vi "eventHandler.vi"(8 "error in (no error)":errorcluster, 9 ":HWControllerEvents":refnum<class "HWControllerEvents.lvclass">, 10 "ExperimentControlEvents":refnum<class "ExperimentControlEvents.lvclass">, 11 "ExperimentControl in":refnum<class "ExperimentControl.lvclass">) -> (0 "error out":errorcluster, 3 "ExperimentControl out":refnum<class "ExperimentControl.lvclass">)   [LabVIEW 2009, in "Views.lvlib" / "ExperimentControl.lvlib" / "ExperimentControl.lvclass"]
uses:
  ExperimentControl.lvclass
  Events/ExperimentControlEvents.lvclass
  Hal/HWController/HWControllerEvents/HWControllerEvents.lvclass
  ExperimentControl.lvclass/ExperimentControl.ctl
  Events/Event.lvclass
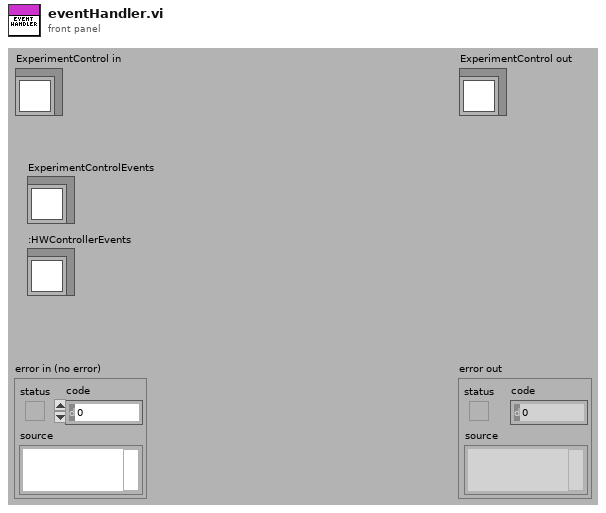
[diagram p1: front panel]
types:
  T1 = enum16{"Ready", "Compiling", "Configured", "Running", "Stopping", "Unresolved Error"}
  T2 = enum16{"close", "stopRunning", "runSingleScript", "runExperiment", "runExperimentScript", "Unregistered", "hasStopped"}
  T3 = cluster{"Array":path[], "Enum":enum16{"runListOnce", "loopOverList"}}
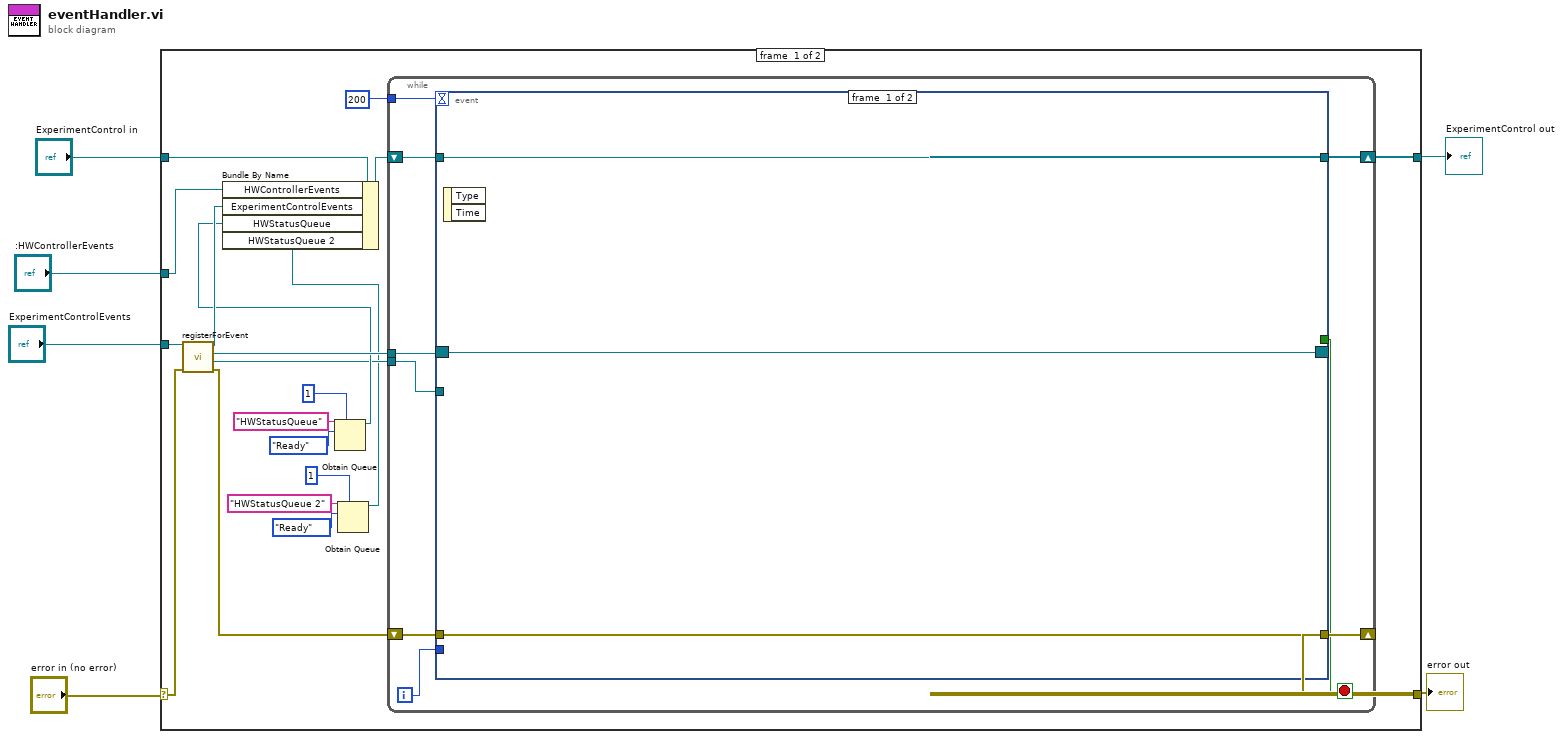
[diagram p0: block diagram]
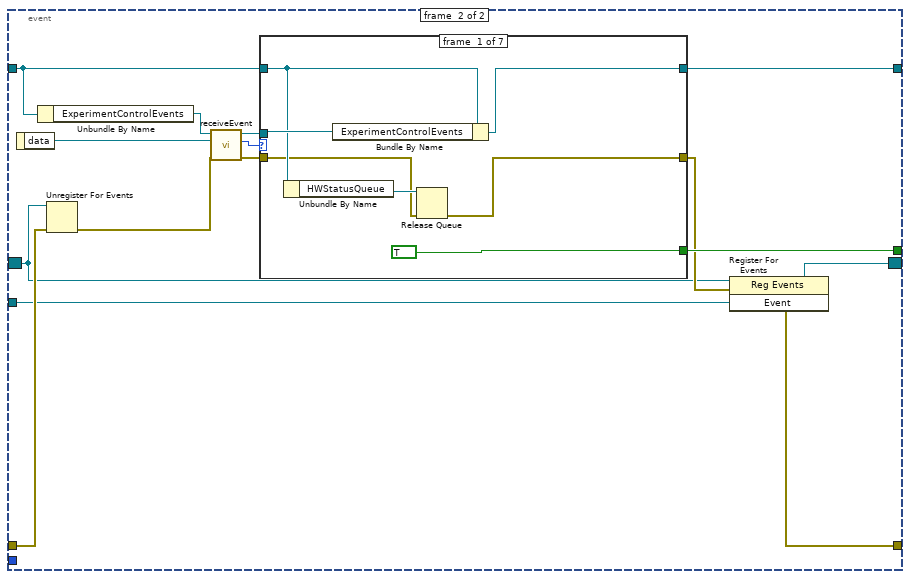
[diagram p2: hidden frame]
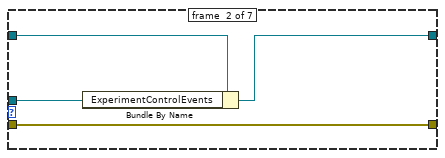
[diagram p3: hidden frame]
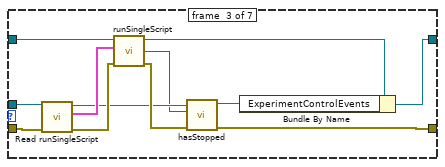
[diagram p4: hidden frame]
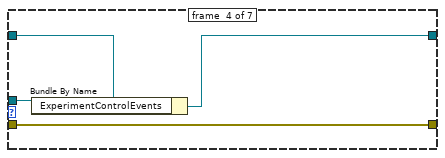
[diagram p5: hidden frame]
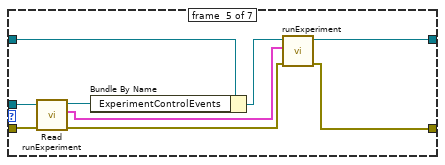
[diagram p6: hidden frame]
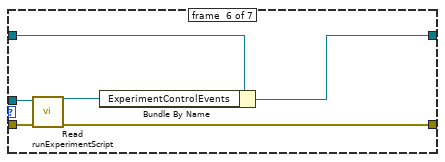
[diagram p7: hidden frame]
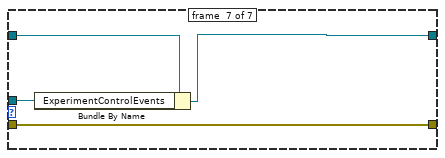
[diagram p8: hidden frame]
diagram:
  n1 = case shown="No Error" "error in (no error)" {
    selector: "error in (no error)" -> [w21 w101]
    tunnel: [w25 w101] -> w5
    tunnel: [w26 w100] -> w1
    tunnel: "ExperimentControl in" -> [w24 w100]
    tunnel: "ExperimentControlEvents" -> [w22 _]
    tunnel: ":HWControllerEvents" -> [w17 _]
    frame #0 {
      n2 = call "registerForEvent.vi"("error in (no error)"=w21, "Event in"=w22) -> ("error out"=w19:errorcluster, "Event"=w11:refnum<user-event>, "Event Registration Refnum"=w20:refnum<event-registration>, "Event out"=w18:refnum<class "ExperimentControlEvents.lvclass">)  [unwired: 6 in]
      n3 = Obtain Queue(max queue size (-1, unlimited)=1, name (unnamed)="HWStatusQueue", element data type=T1."Ready" ("status")) -> (queue out=w12:refnum<queue>)  [unwired: 2 in, 2 out]
      n4 = Obtain Queue(max queue size (-1, unlimited)=1, name (unnamed)="HWStatusQueue 2", element data type=T1."Ready" ("status")) -> (queue out=w7:refnum<queue>)  [unwired: 2 in, 2 out]
      n5 = Bundle By Name(cluster=w24, "HWControllerEvents"=w17, "ExperimentControlEvents"=w18, "HWStatusQueue"=w12, "HWStatusQueue 2"=w7) -> (w23:refnum<class "ExperimentControl.lvclass">)
      n6 = while {
        shift-right: [w32] -> w25
        shift-left: w19 -> [w33]
        shift-right: [w35] -> w26
        shift-left: w23 -> [w34]
        tunnel: w20 -> [w31]
        tunnel: 200 -> [w27]
        tunnel: w11 -> [w28]
        i -> [w29]
        stop <- w30 stop-if-true
        n7 = event shown="[1] <Event>: User Event" {
          selector: w31 -> [w36 w39]
          dyn-events: [w36 w41] -> _
          timeout: w27 -> [_ _]
          tunnel: [w38 w44] -> w35
          tunnel: w34 -> [w38 w48]
          tunnel: w33 -> [w37 w46]
          tunnel: [w37 w40] -> w32
          tunnel: [_ w50] -> w30
          tunnel: w29 -> [_ _]
          tunnel: w28 -> [_ w43]
          event #0 {
            n8 = event-data() -> ()  [unwired: 1 in, 2 out]
          }
          event #1 {
            n9 = event-data() -> ("data"=w52:refnum<class>)  [unwired: 1 in]
            n10 = Unbundle By Name(w48) -> ("ExperimentControlEvents"=w53:refnum<class "ExperimentControlEvents.lvclass">)
            n11 = Unregister For Events(event registration refnum=w39, error in=w46) -> (error out=w45:errorcluster)
            n12 = call "receiveEvent.vi"("error in (no error)"=w45, "data"=w52, "ExperimentControlEvents in"=w53) -> ("error out"=w49:errorcluster, "Enum"=w51:T2, "ExperimentControlEvents out"=w47:refnum<class "ExperimentControlEvents.lvclass">)  [unwired: 6 in]
            n13 = case shown="\"hasStopped\"" w51 {
              tunnel: w47 -> [w58 w62 w74 w79 w89 w92 w98]
              tunnel: [TRUE _ _ _ _ _ _] -> w50
              tunnel: w49 -> [w55 w61 w73 w80 w88 w93 w99]
              tunnel: [w54 w61 w72 w80 w82 w90 w99] -> w42
              tunnel: w48 -> [w57 w64 w70 w78 w86 w95 w97]
              tunnel: [w59 w63 w66 w77 w84 w94 w96] -> w44
              frame #0 {
                n14 = Unbundle By Name(w57) -> ("HWStatusQueue"=w56:refnum<queue>)
                n15 = Bundle By Name(cluster=w57, "ExperimentControlEvents"=w58) -> (w59:refnum<class "ExperimentControl.lvclass">)
                n16 = Release Queue(queue=w56, error in (no error)=w55) -> (error out=w54:errorcluster)  [unwired: 1 in, 2 out]
              }
              frame #1 {
                n17 = Bundle By Name(cluster=w64, "ExperimentControlEvents"=w62) -> (w63:refnum<class "ExperimentControl.lvclass">)
              }
              frame #2 {
                n18 = call "Read runSingleScript.vi"("error in (no error)"=w73, "ExperimentControlEvents in"=w74) -> ("error out"=w76:errorcluster, "runSingleScript"=w75:cluster{"Path":path, "HWLoop":bool}, "ExperimentControlEvents out"=w69:refnum<class "ExperimentControlEvents.lvclass">)  [unwired: 7 in]
                n19 = call "runSingleScript.vi"("error in (no error)"=w76, "runSingleScript"=w75, "ExperimentControl in"=w70) -> ("error out"=w71:errorcluster, "stoppedByUser"=w65:bool, "ExperimentControl out"=w67:refnum<class "ExperimentControl.lvclass">)  [unwired: 5 in, 1 out]
                n20 = call "hasStopped.vi"("error in (no error)"=w71, "stoppedByUser"=w65, "ExperimentControlEvents in"=w69) -> ("error out"=w72:errorcluster, "ExperimentControlEvents out"=w68:refnum<class "ExperimentControlEvents.lvclass">)  [unwired: 7 in]
                n21 = Bundle By Name(cluster=w67, "ExperimentControlEvents"=w68) -> (w66:refnum<class "ExperimentControl.lvclass">)
              }
              frame #3 {
                n22 = Bundle By Name(cluster=w78, "ExperimentControlEvents"=w79) -> (w77:refnum<class "ExperimentControl.lvclass">)
              }
              frame #4 {
                n23 = call "Read runExperiment.vi"("error in (no error)"=w88, "ExperimentControlEvents in"=w89) -> ("error out"=w83:errorcluster, "runExperiment"=w81:T3, "ExperimentControlEvents out"=w87:refnum<class "ExperimentControlEvents.lvclass">)  [unwired: 7 in]
                n24 = Bundle By Name(cluster=w86, "ExperimentControlEvents"=w87) -> (w85:refnum<class "ExperimentControl.lvclass">)
                n25 = call "runExperiment.vi"("error in (no error)"=w83, "runExperiment"=w81, "ExperimentControl in"=w85) -> ("error out"=w82:errorcluster, "ExperimentControl out"=w84:refnum<class "ExperimentControl.lvclass">)  [unwired: 7 in]
              }
              frame #5 {
                n26 = call "Read runExperimentScript.vi"("error in (no error)"=w93, "ExperimentControlEvents in"=w92) -> ("error out"=w90:errorcluster, "ExperimentControlEvents out"=w91:refnum<class "ExperimentControlEvents.lvclass">)  [unwired: 7 in, 1 out]
                n27 = Bundle By Name(cluster=w95, "ExperimentControlEvents"=w91) -> (w94:refnum<class "ExperimentControl.lvclass">)
              }
              frame #6 {
                n28 = Bundle By Name(cluster=w97, "ExperimentControlEvents"=w98) -> (w96:refnum<class "ExperimentControl.lvclass">)
              }
            }
            n29 = register-events(reference=w39, error in=w42, w43) -> (reference out=w41:refnum<event-registration>, error out=w40:errorcluster)
          }
        }
      }
    }
    frame #1 {
    }
  }
  "error out" <- w5
  "ExperimentControl out" <- w1
